vi "Configure Unit of Current.vi"(8 "error in (no error)":errorcluster, 10 "Unit (0: Amps)":u16(ring), 11 "VISA resource name":refnum<visa-resource-name>) -> (0 "error out":errorcluster, 3 "VISA resource name out":refnum<visa-resource-name>)   [LabVIEW 2018, in "Keithley 2450.lvlib"]
doc: "This VI describes the units of measurement that are displayed on the front panel of the instrument and\nstored in the reading buffer."
uses:
  <instrlib>/Keithley 2450/Keithley 2450.lvlib
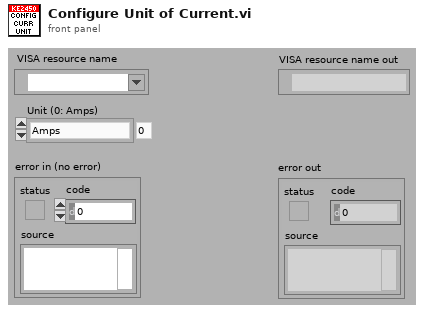
[diagram p1: front panel]
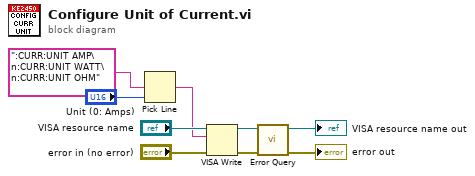
[diagram p0: block diagram]
diagram:
  n1 = Pick Line(multi-line string=":CURR:UNIT AMP\n:CURR:UNIT WATT\n:CURR:UNIT OHM" ("Function"), line index="Unit (0: Amps)") -> (output string=w1:string)  [unwired: 1 out]
  n2 = VISA Write(VISA resource name="VISA resource name", write buffer=w1, error in (no error)="error in (no error)") -> (VISA resource name out=w3:refnum<visa-resource-name>, error out=w2:errorcluster)  [unwired: 1 out]
  n3 = call <instrlib>:"Error Query.vi"("error in (no error)"=w2, "VISA resource name"=w3) -> ("error out"=→"error out":errorcluster, "VISA resource name out"=→"VISA resource name out":refnum<visa-resource-name>)  [unwired: 8 out]
